vi "Arrange Components.vi"(7 "Decos":refnum<vi>[](array[refnum]), 8 "error in (no error)":errorcluster, 11 "ControlArray":refnum<class "ControlArray.lvclass">) -> (0 "error out":errorcluster)   [LabVIEW 2020, in "Control Array.lvlib" / "ControlArray.lvclass"]
uses:
  ControlArray.lvclass
  ControlArray.lvclass/ControlArray.ctl
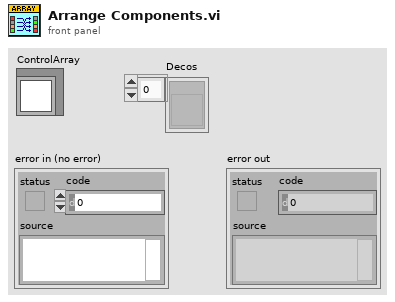
[diagram p1: front panel]
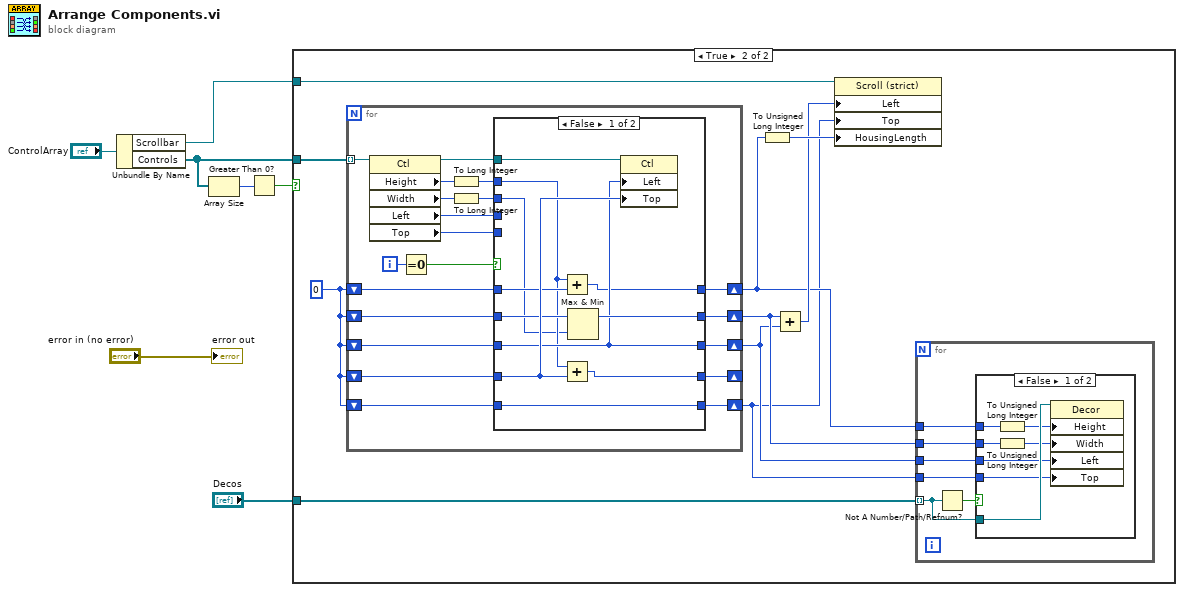
[diagram p0: block diagram]
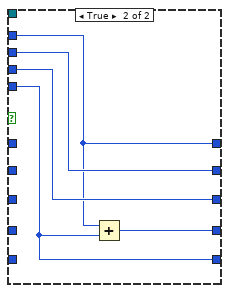
[diagram p4: hidden frame]
diagram:
  n1 = Unbundle By Name("ControlArray") -> ("Scrollbar"=w2:refnum<vi>, "Controls"=w1:refnum<vi>[])
  n2 = Array Size(array=w1) -> (size(s)=w7:i32)
  n3 = Greater Than 0?(x=w7) -> (x > 0?=w6:bool)
  n4 = case shown="True" w6 {
    tunnel: w1 -> [_ w17]
    tunnel: w2 -> [_ w16]
    tunnel: "Decos" -> [_ w13]
    frame False {
    }
    frame True {
      w15 = 0
      n5 = for {
        tunnel: w17 -> [w48] mode=indexing
        shift-right: [w39] -> w11
        shift-left: w15 -> [w42]
        shift-right: [w37] -> w10
        shift-left: w15 -> [w41]
        shift-right: [w38] -> w9
        shift-left: w15 -> [w40]
        shift-right: [w33] -> _
        shift-left: w15 -> [w34]
        shift-right: [w32] -> w8
        shift-left: w15 -> [w31]
        i -> [w50]
        n6 = property class="Ctl"(reference=w48) -> (reference out=w43:refnum<vi>, "Height"=w47:u32, "Width"=w46:u32, "Left"=w45:i32, "Top"=w44:i32)  [unwired: 1 in, 1 out]
        n7 = Equal To 0?(x=w50) -> (x = 0?=w49:bool)
        n8 = To Long Integer(number=w47) -> (32bit integer=w36:i32)
        n9 = To Long Integer(number=w46) -> (32bit integer=w35:i32)
        n10 = case shown="False" w49 {
          tunnel: w36 -> [w54 w64]
          tunnel: w35 -> [w52 w66]
          tunnel: w45 -> [_ w65]
          tunnel: w44 -> [_ w62]
          tunnel: w43 -> [w61 _]
          tunnel: w42 -> [w55 _]
          tunnel: w41 -> [w59 _]
          tunnel: w40 -> [w56 _]
          tunnel: [w53 w64] -> w39
          tunnel: [w56 w65] -> w38
          tunnel: [w58 w66] -> w37
          tunnel: w34 -> [w60 _]
          tunnel: [w57 w63] -> w33
          tunnel: [w51 w62] -> w32
          tunnel: w31 -> [w51 _]
          frame False {
            n11 = Add(x=w54, y=w55) -> (x+y=w53:i32)
            n12 = Add(x=w54, y=w60) -> (x+y=w57:i32)
            n13 = Max & Min(x=w59, y=w52) -> (max(x,y)=w58:i32)  [unwired: 1 out]
            n14 = property class="Ctl"(reference=w61, "Left"=w56, "Top"=w60) -> ()  [unwired: 1 in, 2 out]
          }
          frame True {
            n15 = Add(x=w64, y=w62) -> (x+y=w63:i32)
          }
        }
      }
      n16 = To Unsigned Long Integer(number=w11) -> (unsigned 32bit integer=w14:u32)
      n17 = Add(x=w10, y=w9) -> (x+y=w12:i32)
      n18 = property class="Scroll (strict)"(reference=w16, "Left"=w12, "Top"=w8, "HousingLength"=w14) -> ()  [unwired: 1 in, 2 out]
      n19 = for {
        tunnel: w13 -> [w22] mode=indexing
        tunnel: w11 -> [w21]
        tunnel: w9 -> [w20]
        tunnel: w8 -> [w19]
        tunnel: w10 -> [w18]
        n20 = Not A Number/Path/Refnum?(number/path/refnum=w22) -> (NaN/Path/Refnum?=w23:bool)
        n21 = case shown="False" w23 {
          tunnel: w22 -> [w30 _]
          tunnel: w21 -> [w29 _]
          tunnel: w18 -> [w28 _]
          tunnel: w20 -> [w27 _]
          tunnel: w19 -> [w26 _]
          frame False {
            n22 = To Unsigned Long Integer(number=w29) -> (unsigned 32bit integer=w25:u32)
            n23 = To Unsigned Long Integer(number=w28) -> (unsigned 32bit integer=w24:u32)
            n24 = property class="Decor"(reference=w30, "Height"=w25, "Width"=w24, "Left"=w27, "Top"=w26) -> ()  [unwired: 1 in, 2 out]
          }
          frame True {
          }
        }
      }
    }
  }
  "error out" <- "error in (no error)"
